vi "Dashboard Main.vi"() -> ()   [LabVIEW 2016]
uses:
  <vilib>/event_ctls.llb/eventvkey.ctl
  <vilib>/Utility/config.llb/NI_LVConfig.lvlib
  <vilib>/Utility/config.llb/Write Key (I32).vi
  <vilib>/Rock Robotics/WPI/Dashboard/WPI_DashboardLogging Global.vi
  <vilib>/Utility/config.llb/Write Key (String).vi
  <vilib>/Rock Robotics/Network Tables/NT Read Numeric Array.vi
  <vilib>/Utility/miscctls.llb/LVRowAndColumnTypeDef.ctl
  <vilib>/Instr/_visa.llb/VISA Configure Serial Port (Instr).vi
panel:
  in  "TCP":refnum<k5>
  in  "Rec Mode":enum32{"Stop", "Record", "Playback"}(radio)
  in  "Vision":u16(ring) items=["Camera Off", "USB Camera SW", "USB Camera HW", "IP Camera"]
  out "Camera IP":string
  out "Image Message":string="Timeout in Camera Communications"
  in  "Dashboard Tab":T1(tab)
  in  "Select Auto":string(combo)
  out "NT Connection":bool
  in  "Camera Settings":T2={"Frame Rate"=30, "Compression"=30, "Size"=1} {"Frame Rate" scale=1.0..30.0; "Size" items=["640x480", "320x240", "160x120"]}
  out "MotorChart R":cluster{"Numeric":dbl, "Numeric":dbl}(graph)
  out "MotorChart L":T3(graph)
  out "MotorSliders R":cluster{"MotorSlide1":dbl, "MotorSlide2":dbl} {"MotorSlide2" scale=-1.0..1.0 scale format="%#_2e"; "MotorSlide1" scale=-1.0..1.0 scale format="%#_2e"}
  out "MotorSliders L":T4 {"MotorSlide4 2" scale=0.0..14.0 scale format="%#_2e"; "MotorSlide2" scale=-1.0..1.0 scale format="%#_2e"; "MotorSlide1" scale=-1.0..1.0 scale format="%#_2e"}
  out "Gyro":dbl(knob) scale=0.0..360.0
  out "JS1 Z":dbl(slide) scale=-1.0..1.0 scale format="%#_2e"
  out "JS1 Graph":cluster{"X":dbl, "Y":dbl}[](graph)
  out "JS1 Buttons":T5
  out "JS2 Z":dbl(slide) scale=-1.0..1.0 scale format="%#_2e"
  out "JS2 Graph":cluster{"X":dbl, "Y":dbl}[](graph)
  out "JS2 Buttons":T5
  out "Mode":T6(ring)=enum."Auto Disabled"
  in  "DB Camera Config":bool
  out "fps":dbl format="%#.1g"
  out "Mbps":dbl format="%#.1g"
  out "Mbps LED":bool
  in  "DB/String 9":string
  in  "DB/String 8":string
  in  "DB/String 7":string
  in  "DB/String 6":string
  in  "DB/String 5":string
  in  "DB/String 4":string
  in  "DB/String 3":string
  in  "DB/String 2":string
  in  "DB/String 1":string
  in  "DB/String 0":string
  in  "DB/Slider 0":dbl(slide) scale=0.0..5.0
  in  "DB/Slider 1":dbl(slide) scale=0.0..5.0
  in  "DB/Slider 2":dbl(slide) scale=0.0..5.0
  in  "DB/Slider 3":dbl(slide) scale=0.0..5.0
  out "DB/LED 3":bool
  out "DB/LED 2":bool
  out "DB/LED 1":bool
  out "DB/LED 0":bool
  in  "DB/Button 3":bool
  in  "DB/Button 2":bool
  in  "DB/Button 1":bool
  in  "DB/Button 0":bool caption="New Name"
  out "Boolean":bool
  out "Gauge 2":u8(knob) scale=0.0..255.0
  out "Gauge":u8(knob) scale=0.0..255.0
  out "Boolean 3":bool
  in  "Boolean 2":bool
  out "String 2":string
  out "String":string
  in  "Boolean 4":bool
  out "Boolean 5":bool
  in  "Test Slider":dbl(slide) scale=0.0..100.0 scale format="%#_3g"
  in  "On/Off":bool caption="Solenoid"
  in  "Test Name":u16(ring) items=["Select the test to run..."]
  in  "Test Tree":string(tree)
  in  "Motor":cluster{"Value":dbl, "Enable":bool} {"Value" scale=-1.0..1.0 scale format="%#_3g"}
  out "Progress":T7 {"Test Progress" scale=0.0..100.0}
  in  "Rev/Fwd":cluster{"Forward":bool, "Reverse":bool}
  in  "Test Ring":u16(ring) items=["Monochrome", "Color"]
  out "Cmd Status":string
  in  "Execute Command":bool
  in  "Command Params":string[][](table)
  in  "Command Selection":i32(listbox)
  in  "CheckList":i32(listbox)
  out "Tree":string(tree)
  out "Camera Image":T8(plugin-control)
  out "Background":bool
  # "Left"
  # "Front"
  # "Right"
  # "Battery"
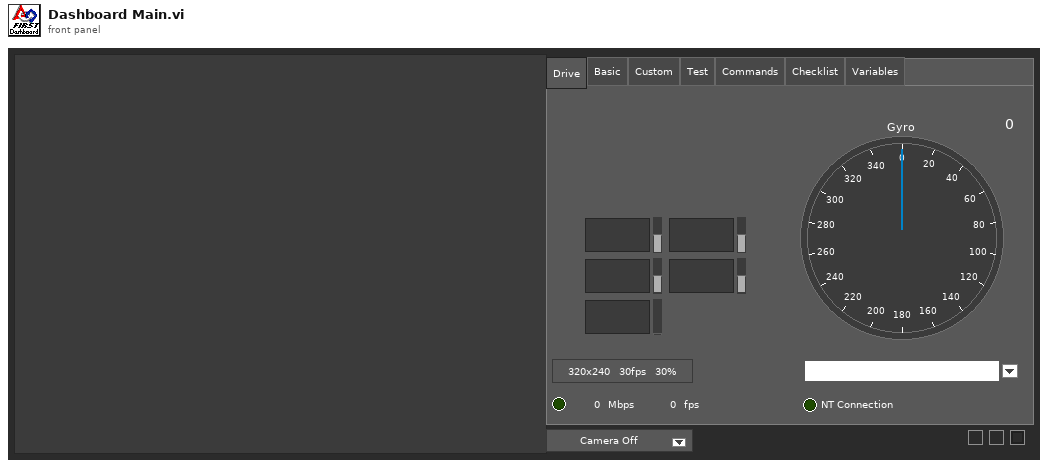
[diagram p1: front panel]
types:
  T1 = enum32{"Drive", "Basic", "Custom", "Test", "Commands", "Checklist", "Variables"}
  T2 = cluster{"Frame Rate":i32, "Compression":i32, "Size":u16}
  T3 = cluster{"Numeric":dbl, "Numeric":dbl, "Battery V":dbl}
  T4 = cluster{"MotorSlide1":dbl, "MotorSlide2":dbl, "MotorSlide4 2":dbl}
  T5 = cluster{bool, bool, bool, bool, bool, bool, bool, bool, bool, bool, bool, bool}
  T6 = enum8{"Tele-Op Disabled", "Tele-Op Enabled", "Auto Disabled", "Auto Enabled", "Test Disabled", "Test Enabled", "Disconnected", "No Code", "E-Stop"}
  T7 = cluster{"Test Progress":u8, "Test Progress Text":string}
  T8 = typedef "IMAQ Image.ctl" = refnum<image>
  T9 = cluster{"IDs":cluster{"RPC field ID":u16, "Unique ID":u16}, "String":string}
  T10 = enum32{"Drive", "Basic", "Custom", "Test", "Checklist", "Variables"}
  T11 = typedef "Image Type" = u32
  T12 = cluster{"Error Strings":string, "Disable Counts":cluster{u16, u16}, "Rail Faults":cluster{u16, u16, u16}, "Robot IP":string, "DB Mode":u8, "Event Info":cluster{"Name":string, "Type":u8, "Number":u16, "Replay":u8}}
  T13 = cluster{"Storage":cluster{"Disk Free":u64, "RAM Block":u32, "RAM free":u32}, "CPU Utilization":cluster{"CPU % ISR":sgl, "CPU % Time Crit":sgl, "CPU % Timed Str":sgl, "CPU % High":sgl, "CPU % Above":sgl, "CPU % Normal":sgl, "CPU % Low":sgl}, "CAN":cluster{"% Bus Utilization":sgl, "Bus Off Cnt":u32, "TX_FIFO Full Cnt":u32, "Receive Error Cnt":u8, "Transmit Error Cnt":u8}, "HID":cluster{"HID Outputs":u32, "Rumble Low":u16, "Rumble High":u16}[]}
  T14 = cluster{"Status bits":cluster{"Test Mode":bool, "Autonomous":bool, "Enabled":bool, "Code Start":bool, "Brownout":bool, "Reserved 2":bool, "Reserved 3":bool, "E-Stop":bool}, "Code Trace":cluster{"Disabled":bool, "TeleOp":bool, "Auto":bool, "Test":bool}, "Controller Type":enum16{"unknown", "cRIO", "roboRio"}, "Code?":enum16{"unknown", "noCode", "code"}, "Battery V":dbl}
  T15 = cluster{"Control Bits":cluster{"TestMode":bool, "Autonomous":bool, "Enabled":bool, "FMS Present":bool, bool, bool, bool, "E-Stop":bool}, "Team Station ":u8, "Countdown":sgl, "Joystick Values":cluster{"Axes":dbl[], "Buttons":bool[], "POVs":i16[]}[]}
  T16 = cluster{"Axes":dbl[], "Buttons":bool[], "POVs":i16[]}[]
  T17 = cluster{"Axes":dbl[], "Buttons":bool[], "POVs":i16[]}
  T18 = cluster{"Buttons[0]":bool, "Buttons[1]":bool, "Buttons[2]":bool, "Buttons[3]":bool, "Buttons[4]":bool, "Buttons[5]":bool, "Buttons[6]":bool, "Buttons[7]":bool, "Buttons[8]":bool, "Buttons[9]":bool, "Buttons[10]":bool, "Buttons[11]":bool}
  T19 = cluster{"Camera Image":refnum<vi>, "Dashboard Tab":refnum<vi>, "Background":refnum<vi>, "Vision":refnum<vi>, "Rec Mode":refnum<vi>, "Test Slider":refnum<vi>, "On/Off ":refnum<vi>, "Test Ring":refnum<vi>, "Rev/Fwd":refnum<vi>, "Test Name":refnum<vi>, "Motor":refnum<vi>, "Progress":refnum<vi>, "CheckList":refnum<vi>, "Tree":refnum<vi>, "Test Tree":refnum<vi>, "Command Params":refnum<vi>, "Command Selection":refnum<vi>, "Execute Command":refnum<vi>, "Cmd Status":refnum<vi>}
  T20 = typedef "NI_LVConfig.lvlib/Config Data RefNum.ctl" = refnum<k1>
  T21 = cluster{"Operation":enum16{"Update", "Clear"}, "Color Box":u32}[]
  T22 = typedef "eventvkey.ctl" = enum16{"ASCII", "Enter", "Return", "Shift", "Ctrl", "Alt", "Cmd", "Opt", "Caps", "NumLock", "Clear", "Break", "Up", "Down", "Left", "Right", "Insert", "Delete", "Home", "End", "PageUp", "PageDown", "Escape", "Help", "Pause", "ScrollLock", "F1", "F2", "F3", "F4", "F5", "F6", "F7", "F8", "F9", "F10", "F11", "F12", "F13", "F14", "F15", "F16", "F17", "F18", "F19", "F20", "F21", "F22", "F23", "F24", "Play", "VolumeUp", "VolumeDown", "Mute", "Two Byte Char"}
  T23 = cluster{"Image Size":bool, "Image Type":bool, "Pixel Value":bool, "ROI Information":bool, "Zoom Factor":bool}
  T24 = enum8{"Enabled", "Disabled", "Disabled and Grayed Out"}
  T25 = cluster{"Operation":enum16{"Update", "Clear"}, "Color Box":u32}
  T26 = typedef "LVRowAndColumnTypeDef.ctl" = cluster{"Row":i32, "Column":i32}
  T27 = cluster{"Shift":bool, "Ctrl":bool, "Alt":bool, "Cmd":bool, "Opt":bool}
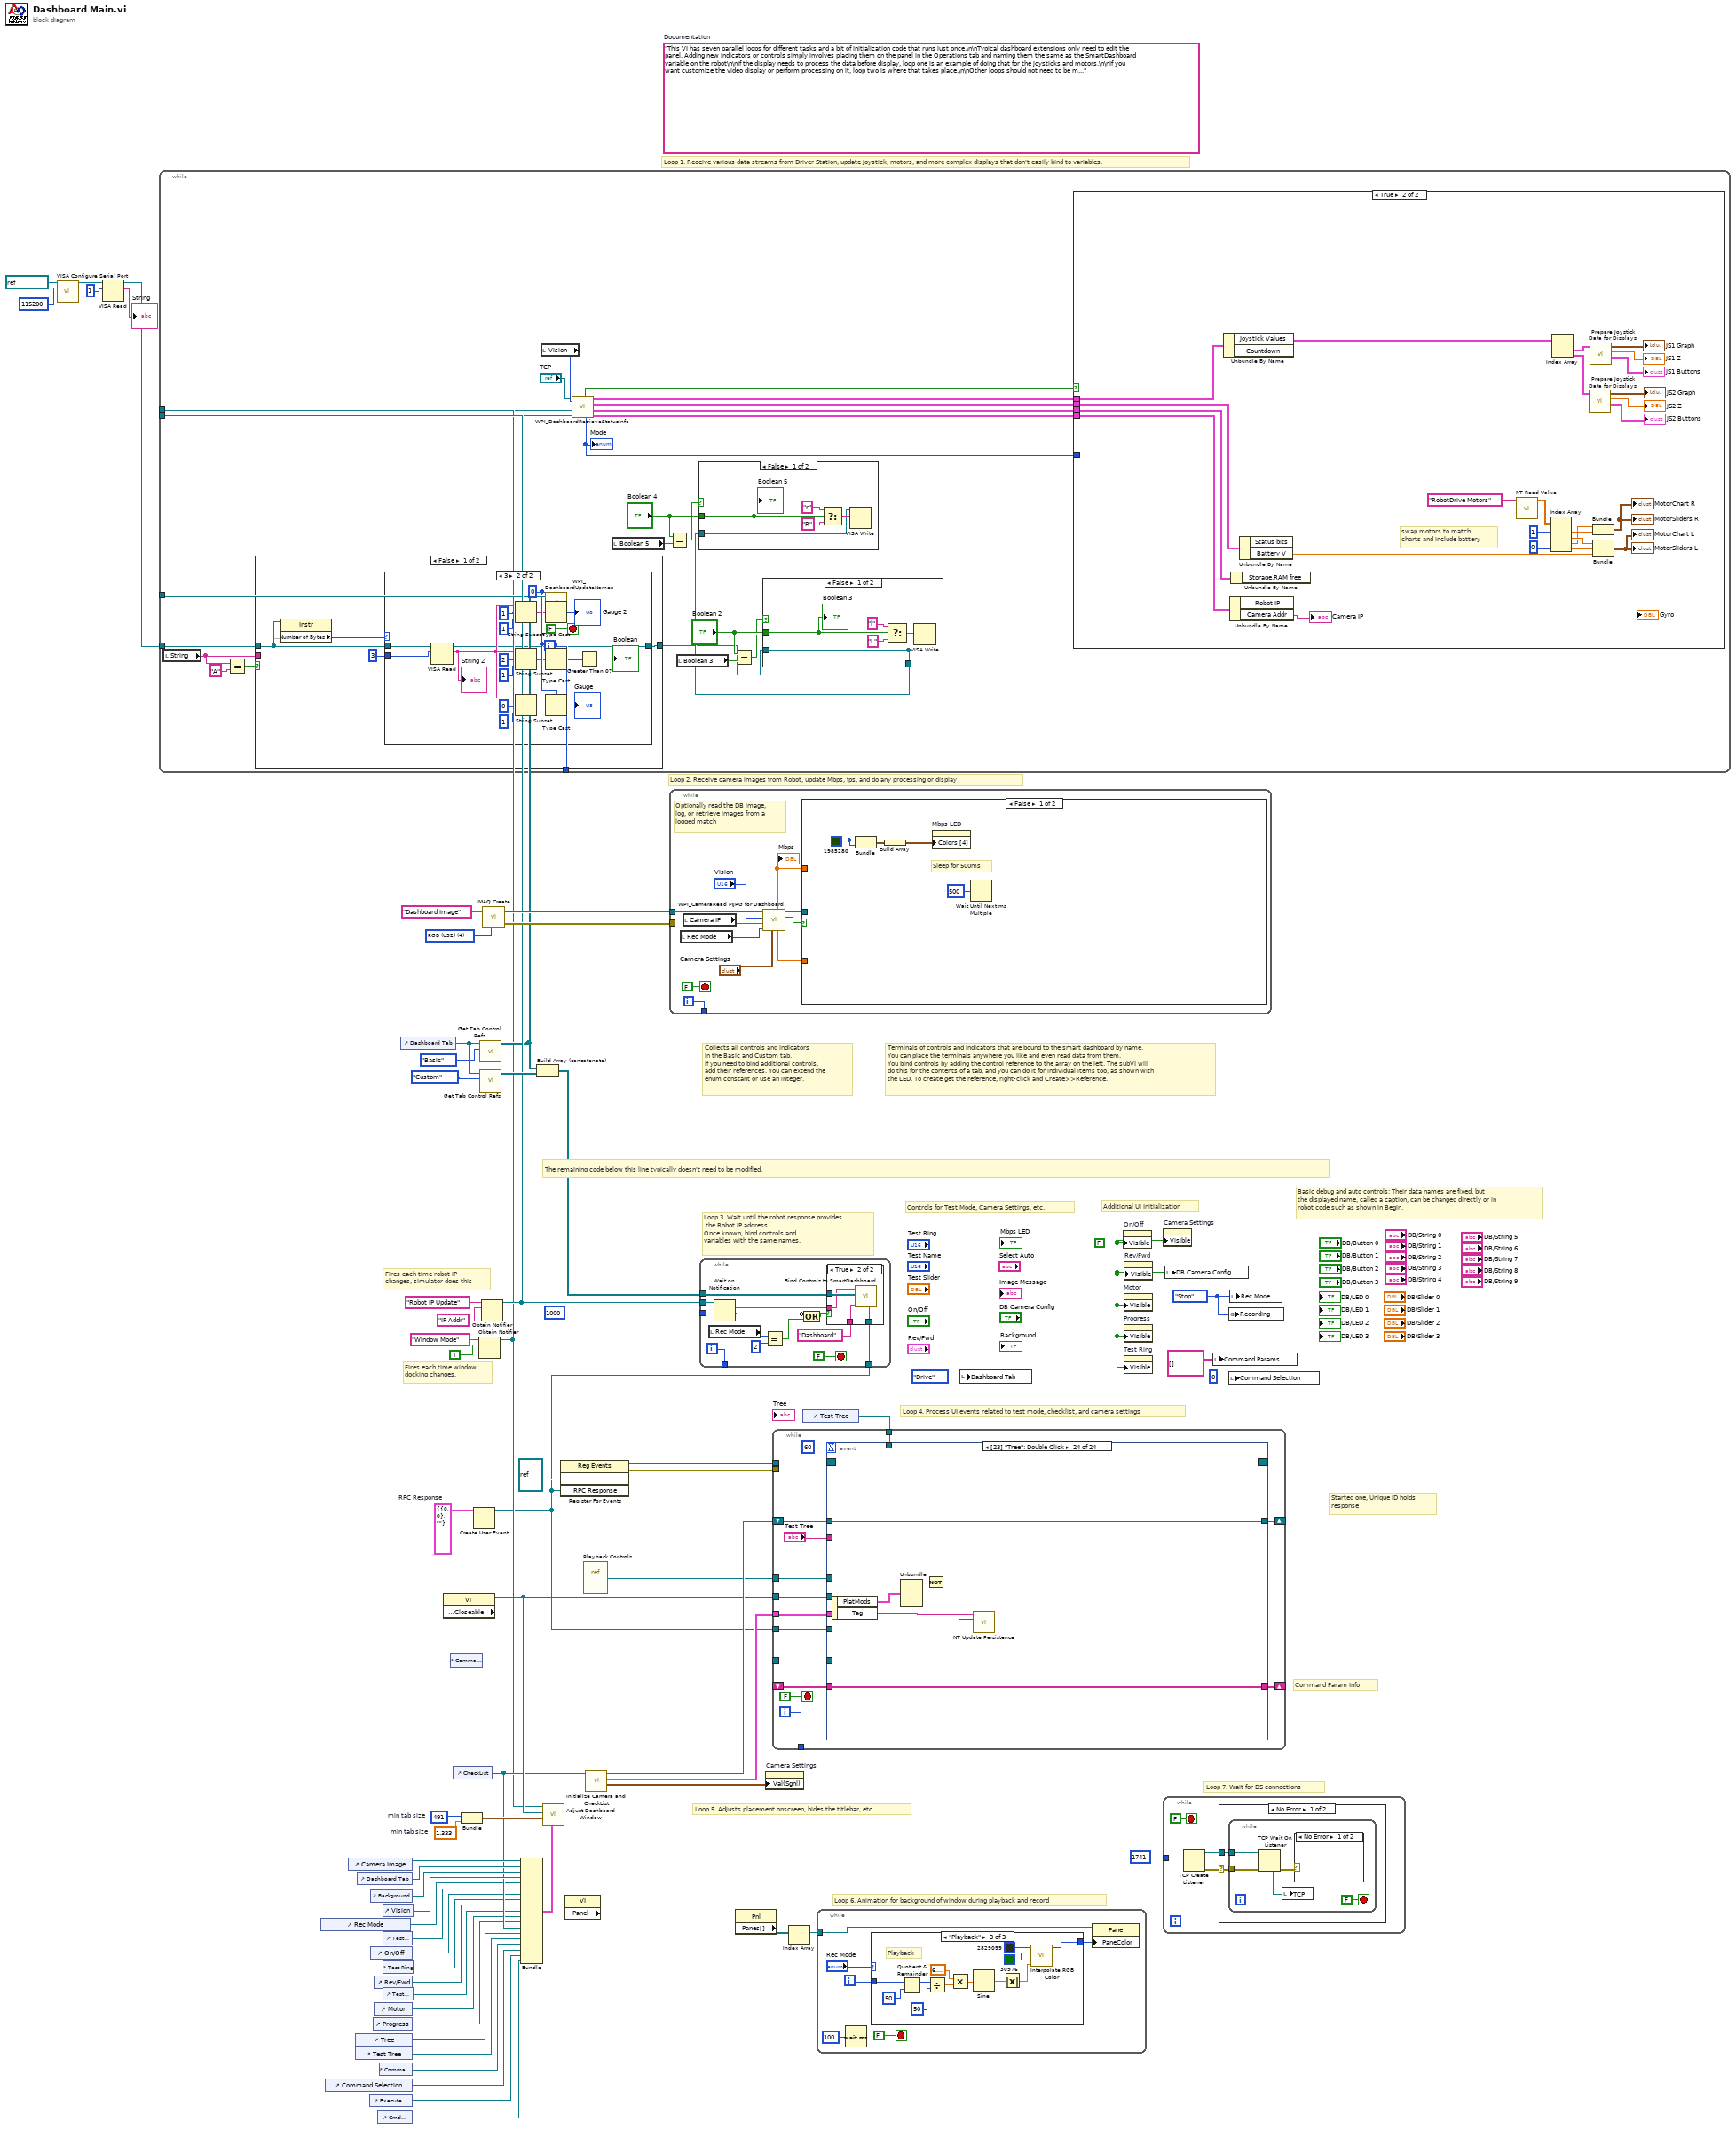
[diagram p0: block diagram]
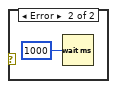
[diagram p2: hidden frame]
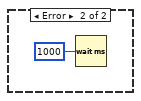
[diagram p3: hidden frame]
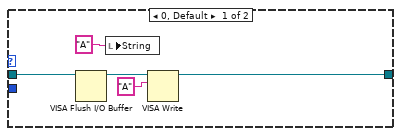
[diagram p6: hidden frame]
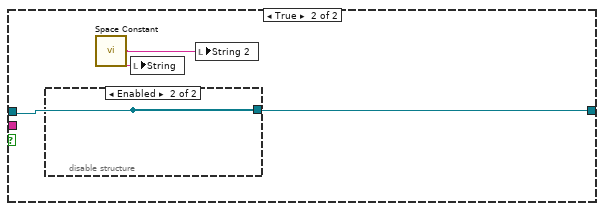
[diagram p7: hidden frame]
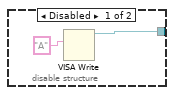
[diagram p8: hidden frame]
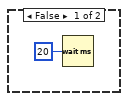
[diagram p9: hidden frame]
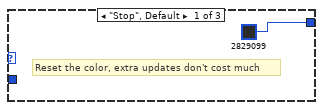
[diagram p10: hidden frame]
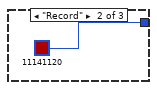
[diagram p11: hidden frame]
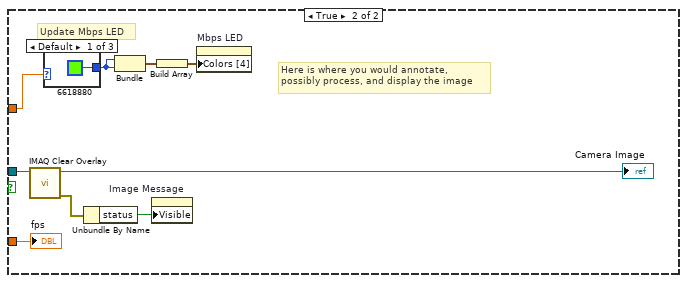
[diagram p13: hidden frame]
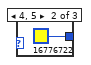
[diagram p14: hidden frame]
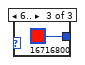
[diagram p15: hidden frame]
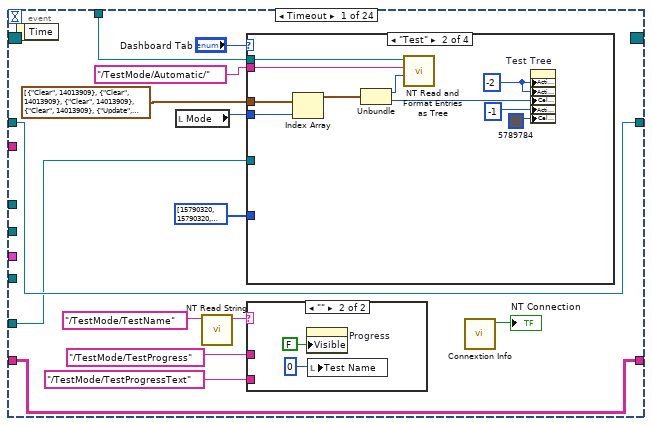
[diagram p16: hidden frame]
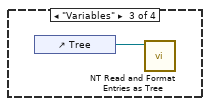
[diagram p18: hidden frame]
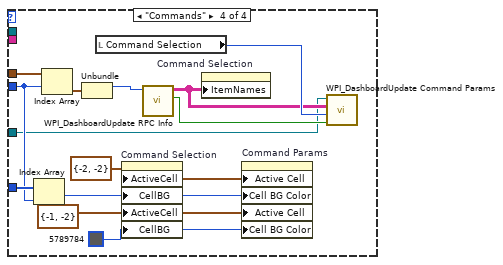
[diagram p19: hidden frame]
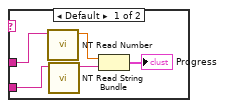
[diagram p20: hidden frame]
diagram:
  w13 = T9 {"IDs"={"RPC field ID"=0, "Unique ID"=0}, "String"=""}  # RPC Response
  w39 = 491  # min tab size
  w38 = 1.333  # min tab size
  w47 = enum32{"Stop", "Record", "Playback"}."Stop" ("Rec Mode")
  w21 = FALSE ("Visible")
  (unwired) "This VI has seven parallel loops for different tasks and a bit of initialization code that runs just once.\n\nTypical dashboard extensions only need to edit the panel. Adding new indicators or controls simply involves placing them on the panel in the Operations tab and naming them the same as the SmartDashboard variable on the robot\n\nIf the display needs to process the data before display, loop one is an example of doing that for the joysticks and motors.\n\nIf you want customize the video display or perform processing on it, loop two is where that takes place.\n\nOther loops should not need to be modified. They are pretty standard, and document the task they perform."  # Documentation
  w67 = T11 4 items=["Grayscale (U8)", "Grayscale (I16)", "Grayscale (SGL)", "Complex (CSG)", "RGB (U32)", "HSL (U32)", "RGB (U64)"] ("Image Type")
  # "Command Param Info"
  # "Started one, Unique ID holds\nresponse"
  # "Loop 7. Wait for DS connections"
  # "Basic debug and auto controls: Their data names are fixed, but\nthe displayed name, called a caption, can be changed directly or in\nrobot code such as shown in Begin."
  # "Controls for Test Mode, Camera Settings, etc."
  # "Additional UI Initialization"
  # "Loop 6. Animation for background of window during playback and record"
  # "Fires each time robot IP\nchanges, simulator does this"
  # "Fires each time window\ndocking changes."
  # "Collects all controls and indicators\nin the Basic and Custom tab.\nIf you need to bind additional controls,\nadd their references. You can extend the\nenum constant or use an integer."
  # "The remaining code below this line typically doesn't need to be modified."
  # "Loop 4. Process UI events related to test mode, checklist, and camera settings"
  # "Terminals of controls and indicators that are bound to the smart dashboard by name.\nYou can place the terminals anywhere you like and even read data from them.\nYou bind controls by adding the control reference to the array on the left. The subVI will\ndo this for the contents of a tab, and you can do it for individual items too, as shown with\nthe LED. To create get the reference, right-click and Create>>Reference."
  # "Loop 3. Wait until the robot response provides\n the Robot IP address.\nOnce known, bind controls and\nvariables with the same names."
  # "Loop 5. Adjusts placement onscreen, hides the titlebar, etc."
  # "Loop 1. Receive various data streams from Driver Station, update joystick, motors, and more complex displays that don't easily bind to variables."
  # "Loop 2. Receive camera images from Robot, update Mbps, fps, and do any processing or display"
  n1 = call-poly "VISA Configure Serial Port"("VISA resource name"=refnum<visa-resource-name> "COM5", "baud rate (9600)"=u32 115200) -> ("VISA resource name out"=w3:refnum<visa-resource-name>)  [unwired: 12 in, 1 out]
  n2 = VISA Read(VISA resource name=w3, byte count=u32 1) -> (VISA resource name out=w1:refnum<visa-resource-name>, read buffer=→"String":string)  [unwired: 1 in, 2 out]
  n3 = control-ref of="Rec Mode"() -> (w27:refnum<vi>)
  n4 = control-ref of="Command Selection"() -> (w12:refnum<vi>)
  n5 = control-ref of="Camera Image"() -> (w42:refnum<vi>)
  n6 = control-ref of="Tree"() -> (w31:refnum<vi>)
  n7 = control-ref of="Test Tree"() -> (w30:refnum<vi>)
  n8 = control-ref of="Dashboard Tab"() -> (w41:refnum<vi>)
  n9 = control-ref of="Execute Command"() -> (w14:refnum<vi>)
  n10 = control-ref of="Background"() -> (w36:refnum<vi>)
  n11 = control-ref of="On/Off"() -> (w25:refnum<vi>)
  n12 = control-ref of="Progress"() -> (w22:refnum<vi>)
  n13 = control-ref of="Rev/Fwd"() -> (w23:refnum<vi>)
  n14 = control-ref of="Motor"() -> (w28:refnum<vi>)
  n15 = control-ref of="Cmd Status"() -> (w8:refnum<vi>)
  n16 = control-ref of="Command Params"() -> (w15:refnum<vi>)
  n17 = control-ref of="Test Slider"() -> (w26:refnum<vi>)
  n18 = control-ref of="Vision"() -> (w40:refnum<vi>)
  n19 = control-ref of="Test Ring"() -> (w24:refnum<vi>)
  n20 = control-ref of="Test Name"() -> (w29:refnum<vi>)
  n21 = control-ref of="Dashboard Tab"() -> (w45:refnum<vi>)
  n22 = property class="VI" props=["Front Panel.Closeable"]() -> (reference out=w46:refnum<vi>)  [unwired: 2 in, 2 out]
  n23 = control-ref of="Command Params"() -> (w7:refnum<vi>)
  n24 = control-ref of="CheckList"() -> (w32:refnum<vi>)
  n25 = Bundle("min tab size"=w39, "min tab size"=w38) -> (w37:cluster{"min tab size":i32, "min tab size":dbl})  [unwired: 1 in]
  n26 = Create User Event(user event datatype=w13) -> (user event=w9:refnum<user-event>)  [unwired: 1 in, 1 out]
  n27 = Obtain Notifier(name (unnamed)="Window Mode", notification data type=TRUE) -> (notifier out=w18:refnum<notifier>)  [unwired: 2 in, 2 out]
  n28 = call <vilib>:"Get Tab Control Refs.vi"("Page Index"=T10."Basic" ("Dashboard Tab"), "TabControl in"=w45) -> ("ControlsOnPage"=w19:refnum<vi>[])  [unwired: 9 in]
  n29 = call <vilib>:"Get Tab Control Refs.vi"("Page Index"=T10."Custom" ("Dashboard Tab"), "TabControl in"=w45) -> ("ControlsOnPage"=w44:refnum<vi>[])  [unwired: 9 in]
  n30 = Obtain Notifier(name (unnamed)="Robot IP Update", notification data type="IP Addr" ("name (unnamed)")) -> (notifier out=w20:refnum<notifier>)  [unwired: 2 in, 2 out]
  n31 = while {
    tunnel: [w91] -> _
    tunnel: w20 -> [w85]
    tunnel: w19 -> [w84]
    tunnel: w18 -> [w80]
    tunnel: w1 -> [w73]
    i -> [w91]
    stop <- FALSE stop-if-true
    n32 = local read "String"() -> (w76:string)
    n33 = Equal?(x=w76, y="A") -> (x = y?=w75:bool)
    n34 = case shown="False" w75 {
      tunnel: w73 -> [w106 w131]
      tunnel: w76 -> [_ _]
      tunnel: [w104 w131] -> w68
      frame False {
        n35 = property class="Instr"(reference=w106) -> ("Serial Settings:Number of Bytes at Serial Port"=w105:u32)  [unwired: 1 in, 2 out]
        n36 = case shown="3" w105 {
          tunnel: u32 3 ("byte count") -> [_ w128]
          tunnel: w106 -> [w111 w127]
          tunnel: [w108 w113] -> w104
          frame 0, Default {
            n37 = VISA Flush I/O Buffer(VISA resource name=w111) -> (VISA resource name out=w109:refnum<visa-resource-name>)  [unwired: 2 in, 1 out]
            n38 = local write "String"("A" ("String")) -> ()
            n39 = VISA Write(VISA resource name=w109, write buffer="A") -> (VISA resource name out=w108:refnum<visa-resource-name>)  [unwired: 1 in, 2 out]
          }
          frame 3 {
            w129 = u8 0
            n40 = VISA Read(VISA resource name=w127, byte count=w128) -> (VISA resource name out=w113:refnum<visa-resource-name>, read buffer=w116:string)  [unwired: 1 in, 2 out]
            "String 2" <- w116
            n41 = String Subset(string=w116, offset (0)=1, length (rest)=1 ("length (rest)")) -> (substring=w115:string)
            n42 = String Subset(string=w116, offset (0)=2, length (rest)=1 ("length (rest)")) -> (substring=w121:string)
            n43 = String Subset(string=w116, offset (0)=0, length (rest)=1 ("length (rest)")) -> (substring=w114:string)
            n44 = Type Cast(type=w129, x=w115) -> (*(type *) &x=→"Gauge 2":u8)
            n45 = Type Cast(type=w129, x=w121) -> (*(type *) &x=w125:u8)
            n46 = Type Cast(type=w129, x=w114) -> (*(type *) &x=→"Gauge":u8)
            n47 = Greater Than 0?(x=w125) -> (x > 0?=→"Boolean":bool)
          }
        }
      }
      frame True {
        n48 = disable-structure shown="Enabled" {
          disable-tunnel: w131 -> [w133 _]
          frame Disabled {
            n49 = VISA Write(VISA resource name=w133, write buffer="A") -> ()  [unwired: 1 in, 3 out]
          }
          frame Enabled {
          }
        }
        n50 = call <vilib>:"Space Constant.vi"() -> ("String"=w132:string)
        n51 = local write "String"(w132) -> ()
        n52 = local write "String 2"(w132) -> ()
      }
    }
    n53 = local read "Vision"() -> (w82:u16)
    n54 = call <vilib>:"WPI_DashboardUpdateNames.vi"("Controls on Tab"=w84) -> ()  [unwired: 11 in]
    n55 = call <vilib>:"WPI_DashboardRetrieveStatusInfo.vi"(7:w82, "Binding Refnum"=w85, "Window Mode Notifier"=w80, "TCP Cnx"="TCP") -> ("Power and Errors"=w86:T12, "Robot Metrics"=w89:T13, "Status Info"=w90:T14, "Control Info"=w87:T15, "Robot Mode"=w83:T6, "Process?"=w88:bool)  [unwired: 2 in]
    "Mode" <- w83
    n56 = local read "Boolean 5"() -> (w70:bool)
    n57 = Equal?(x="Boolean 4", y=w70) -> (x = y?=w71:bool)
    n58 = local read "Boolean 3"() -> (w77:bool)
    n59 = Equal?(x="Boolean 2", y=w77) -> (x = y?=w78:bool)
    n60 = case shown="False" w78 {
      tunnel: "Boolean 2" -> [w100 _]
      tunnel: w68 -> [w98 w103]
      tunnel: [w98 w103] -> w69
      frame False {
        n61 = Select(t="l" ("write buffer"), s=w100, f="L" ("write buffer")) -> (s? t:f=w99:string)
        n62 = VISA Write(VISA resource name=w98, write buffer=w99) -> ()  [unwired: 1 in, 3 out]
        "Boolean 3" <- w100
      }
      frame True {
      }
    }
    n63 = case shown="False" w71 {
      tunnel: "Boolean 4" -> [w95 _]
      tunnel: w69 -> [w93 _]
      frame False {
        n64 = Select(t="r" ("write buffer"), s=w95, f="R" ("write buffer")) -> (s? t:f=w94:string)
        n65 = VISA Write(VISA resource name=w93, write buffer=w94) -> ()  [unwired: 1 in, 3 out]
        "Boolean 5" <- w95
      }
      frame True {
      }
    }
    n66 = case shown="True" w88 {
      tunnel: w90 -> [_ w160]
      tunnel: w89 -> [_ w159]
      tunnel: w87 -> [_ w158]
      tunnel: w86 -> [_ w157]
      tunnel: w83 -> [_ _]
      frame False {
        n67 = Wait (ms)(milliseconds to wait=u32 20) -> ()  [unwired: 1 out]
      }
      frame True {
        # "swap motors to match\ncharts and include battery"
        n68 = Unbundle By Name(w158) -> ("Joystick Values"=w147:T16)  [unwired: 1 out]
        n69 = Unbundle By Name(w157) -> ("Camera Addr"=→"Camera IP":string)  [unwired: 1 out]
        n70 = Unbundle By Name(w159) -> ()  [unwired: 1 out]
        n71 = Unbundle By Name(w160) -> ("Battery V"=w148:dbl)  [unwired: 1 out]
        n72 = call-poly <vilib>:"NT Read Value.vi"("Name"="RobotDrive Motors") -> ("Numeric Array"=w136:dbl[])  [unwired: 9 in, 1 out]
        n73 = Index Array(array=w136, index #1=1, index #4=0) -> (element #1=w152:dbl, element #2=w153:dbl, element #3=w151:dbl, element #4=w156:dbl)  [unwired: 2 in]
        n74 = Index Array(array=w147) -> (element #1=w146:T17, element #2=w141:T17)  [unwired: 2 in]
        n75 = call "Prepare Joystick Data for Displays.vi"("Joystick Values"=w141) -> ("Buttons"=→"JS2 Buttons":T18, "Z Axis"=→"JS2 Z":dbl, "Cartesian Data"=→"JS2 Graph":cluster{"X axis":dbl, "X axis":dbl}[])  [unwired: 8 in]
        n76 = call "Prepare Joystick Data for Displays.vi"("Joystick Values"=w146) -> ("Buttons"=→"JS1 Buttons":T18, "Z Axis"=→"JS1 Z":dbl, "Cartesian Data"=→"JS1 Graph":cluster{"X axis":dbl, "X axis":dbl}[])  [unwired: 8 in]
        n77 = Bundle("Numeric"=w151, "Numeric"=w152) -> (→"MotorChart R" →"MotorSliders R":cluster{"Numeric":dbl, "Numeric":dbl})  [unwired: 1 in]
        n78 = Bundle("Numeric"=w153, "Numeric"=w156, "Battery V"=w148) -> (→"MotorChart L" →"MotorSliders L":T3)  [unwired: 1 in]
      }
    }
  }
  n79 = call "IMAQ Create"("Image Name"="Dashboard Image", "Image Type"=w67) -> ("New Image"=w65:T8, "error out"=w64:errorcluster)  [unwired: 2 in, 1 out]
  n80 = Bundle("Camera Image"=w42, "Dashboard Tab"=w41, "Background"=w36, "Vision"=w40, "Rec Mode"=w27, "Test Slider"=w26, "On/Off"=w25, "Test Ring"=w24, "Rev/Fwd"=w23, "Test Name"=w29, "Motor"=w28, "Progress"=w22, "CheckList"=w32, "Tree"=w31, "Test Tree"=w30, "Command Params"=w15, "Command Selection"=w12, "Execute Command"=w14, "Cmd Status"=w8) -> (w33:T19)  [unwired: 1 in]
  n81 = Build Array (concatenate)(w19, w44) -> (w43:refnum<vi>[])
  n82 = call "Adjust Dashboard Window.vi"("Sizing Refnums"=w33, "Size Constraints"=w37, "VI"=w46, "WIn Mode"=w18) -> ()  [unwired: 8 in]
  n83 = register-events(refnum<vi> refnum, w9) -> (reference out=w51:refnum<event-registration>, error out=w50:errorcluster)  [unwired: 2 in]
  n84 = property class="VI"() -> ("Panel"=w54:refnum<vi>)  [unwired: 2 in, 2 out]
  n85 = vi-ref "Playback Controls.vi"() -> (w52:refnum<vi>)
  n86 = call "Initialize Camera and CheckList.vi"("ListBox in"=w32) -> ("Cluster"=w58:cluster{"value":i32, "value":i32, "index":i32}, "Array"=w59:cluster{string[]}[], "File Refnum"=w57:T20)  [unwired: 8 in]
  n87 = while {
    tunnel: w65 -> [w169]
    tunnel: w64 -> [_]
    tunnel: [w170] -> _
    i -> [w170]
    stop <- FALSE stop-if-true
    # "Optionally read the DB image,\nlog, or retrieve images from a\nlogged match"
    n88 = local read "Rec Mode"() -> (w164:enum32{"Stop", "Record", "Playback"})
    n89 = local read "Camera IP"() -> (w162:string)
    n90 = call <vilib>:"WPI_CameraRead MJPG for Dashboard.vi"("Camera Settings"="Camera Settings", "Rec Mode"=w164, "Robot IP"=w162, "Camera Name"="Vision", "Refnum in"=w169) -> ("Active"=w167:bool, "Refnum out"=w168:T8, "FPS"=w166:dbl, "Bandwidth (Mbps)"=w161:dbl)  [unwired: 3 in]
    "Mbps" <- w161
    n91 = case shown="False" w167 {
      tunnel: w168 -> [_ w179]
      tunnel: w161 -> [_ w178]
      tunnel: w166 -> [_ w176]
      frame False {
        w172 = u32 1985280 ("Color Box")
        # "Sleep for 500ms"
        n92 = Bundle("Color Box"=w172, "Color Box"=w172) -> (w174:cluster{"Color Box":u32, "Color Box":u32})  [unwired: 1 out]
        n93 = Build Array(w174) -> (w173:cluster{"Color Box":u32, "Color Box":u32}[])
        n94 = property on="Mbps LED" class="Bool (strict)"("Colors [4]"=w173) -> ()  [unwired: 2 in, 2 out]
        n95 = Wait Until Next ms Multiple(millisecond multiple=u32 500) -> ()  [unwired: 1 out]
      }
      frame True {
        # "Here is where you would annotate,\npossibly process, and display the image"
        # "Update Mbps LED"
        n96 = call "IMAQ Clear Overlay"("Image"=w179) -> ("error out"=w183:errorcluster, "Image Out"=→"Camera Image":T8)  [unwired: 2 in, 7 out]
        n97 = case shown="Default" w178 {
          tunnel: [u32 6618880 ("Color Box") u32 16776722 ("Color Box") u32 16716800 ("Color Box")] -> w180
          frame Default {
          }
          frame 4, 5 {
          }
          frame 6.. {
          }
        }
        n98 = Unbundle By Name(w183) -> ("status"=w184:bool)
        n99 = Bundle("Color Box"=w180, "Color Box"=w180) -> (w182:cluster{"Color Box":u32, "Color Box":u32})  [unwired: 1 out]
        n100 = property on="Image Message" class="Str"("Visible"=w184) -> ()  [unwired: 2 in, 2 out]
        n101 = Build Array(w182) -> (w181:cluster{"Color Box":u32, "Color Box":u32}[])
        n102 = property on="Mbps LED" class="Bool (strict)"("Colors [4]"=w181) -> ()  [unwired: 2 in, 2 out]
        "fps" <- w176
      }
    }
  }
  n103 = while {
    tunnel: w43 -> [w200]
    tunnel: w20 -> [w198]
    tunnel: [w196] -> _
    tunnel: u32 1000 ("milliseconds to wait") -> [w195]
    tunnel: w9 -> [w188]
    i -> [w196]
    stop <- FALSE stop-if-true
    n104 = local read "Rec Mode"() -> (w191:enum32{"Stop", "Record", "Playback"})
    n105 = Wait on Notification(notifier=w198, timeout in ms (-1)=w195) -> (notification=w197:string, timed out?=w193:bool)  [unwired: 2 in, 2 out]
    n106 = Equal?(x=w191, y=u16 2 ("Rec Mode")) -> (x = y?=w192:bool)
    n107 = Compound Arithmetic op=OR(invert w193, w192) -> (w194:bool)
    n108 = case shown="True" w194 {
      tunnel: w200 -> [_ w204]
      tunnel: w197 -> [_ w203]
      tunnel: "Dashboard" -> [_ w202]
      tunnel: w188 -> [_ w201]
      frame False {
      }
      frame True {
        n109 = call <vilib>:"Bind Controls to SmartDashboard.vi"("RPC ref"=w201, "Client Name"=w202, "Bound Control Refs"=w204, "Server IP Address"=w203) -> ()  [unwired: 8 in]
      }
    }
  }
  n110 = property class="Pnl"(reference=w54) -> ("Panes[]"=w55:refnum<vi>[])  [unwired: 1 in, 2 out]
  n111 = property on="Camera Settings" class="Clust (strict)"("Val(Sgnl)"=w58) -> ()  [unwired: 2 in, 2 out]
  n112 = Index Array(array=w55) -> (element=w53:refnum<vi>)  [unwired: 1 in]
  n113 = control-ref of="Test Tree"() -> (w56:refnum<vi>)
  n114 = while {
    tunnel: w59 -> [w216]
    shift-right: [w215] -> _
    shift-left: w57 -> [w214]
    tunnel: [w213] -> _
    tunnel: w56 -> [w212]
    tunnel: w52 -> [w211]
    tunnel: w51 -> [w210]
    tunnel: w50 -> [_]
    tunnel: w46 -> [w209]
    tunnel: w9 -> [w208]
    tunnel: w7 -> [w207]
    shift-right: [w206] -> _
    shift-left: _ -> [w205]
    i -> [w213]
    stop <- FALSE stop-if-true
    n115 = event shown="[23] \"Tree\": Double Click" {
      selector: w210 -> [_ _ _ _ _ _ _ _ _ _ _ _ _ _ _ _ _ _ _ _ _ _ _ _]
      dyn-events: [_ _ _ _ _ _ _ _ _ _ _ _ _ _ _ _ _ _ w525 _ _ _ _ _] -> _
      timeout: u32 60 ("milliseconds to wait") -> [_ _ _ _ _ _ _ _ _ _ _ _ _ _ _ _ _ _ _ _ _ _ _ _]
      tunnel: w212 -> [w229 _ _ _ _ _ _ _ _ _ _ _ _ _ _ _ _ _ _ _ _ _ _ _]
      tunnel: "Test Tree" -> [_ _ _ _ _ _ _ _ _ _ _ _ _ w488 w497 w500 w505 w514 _ _ _ _ _ _]
      tunnel: w216 -> [_ w267 _ _ _ _ _ _ _ _ _ w450 w481 _ _ _ _ _ _ _ _ _ _ _]
      tunnel: [w226 w266 w370 w376 w386 w390 w396 w408 w416 w422 w435 w449 w474 w487 w495 w499 w504 w513 w527 w543 w545 w553 w564 w569] -> w215
      tunnel: w214 -> [w226 w266 w370 w376 w386 w390 w396 w408 w416 w422 w435 w448 w474 w487 w495 w499 w504 w513 w527 w543 w545 w553 w564 w569]
      tunnel: w211 -> [_ _ _ _ _ _ _ _ _ _ _ _ _ _ _ _ _ _ w528 _ w548 _ _ _]
      tunnel: w209 -> [_ _ _ _ _ _ _ _ _ _ _ _ _ _ _ _ _ _ w523 _ _ _ _ _]
      tunnel: w208 -> [_ _ _ _ _ _ _ _ _ _ _ _ _ _ _ _ _ _ w519 _ _ _ _ _]
      tunnel: w207 -> [w221 _ _ _ _ _ w394 _ _ _ _ _ _ _ _ _ _ _ _ _ _ _ _ _]
      tunnel: [w220 w265 w369 w375 w385 w391 w392 w402 w413 w421 w434 w447 w473 w486 w494 w498 w503 w512 w518 w541 w544 w549 w557 w570] -> w206
      tunnel: w205 -> [w220 w265 w369 w375 w385 w391 w392 _ _ w421 w434 w447 w473 w486 w494 w498 w503 w512 w518 w541 w544 w549 w557 w570]
      event Timeout {
        n116 = event-data() -> ()  [unwired: 1 in, 1 out]
        n117 = local read "Mode"() -> (w223:T6)
        n118 = call <vilib>:"NT Read String.vi"("Name"="/TestMode/TestName") -> ("String"=w232:string)  [unwired: 9 in, 1 out]
        n119 = case shown="\"Test\"" "Dashboard Tab" {
          tunnel: w229 -> [_ w243 _ _]
          tunnel: "/TestMode/Automatic/" ("Name Pattern") -> [_ w242 _ _]
          tunnel: T21 [{"Operation"=enum."Clear", "Color Box"=14013909}, {"Operation"=enum."Clear", "Color Box"=14013909}, {"Operation"=enum."Clear", "Color Box"=14013909}, {"Operation"=enum."Clear", "Color Box"=14013909}, {"Operation"=enum."Update", "Color Box"=14013909}, {"Operation"=enum."Update", "Color Box"=16777215}, {"Operation"=enum."Clear", "Color Box"=14013909}, {"Operation"=enum."Clear", "Color Box"=14013909}, {"Operation"=enum."Clear", "Color Box"=14013909}] -> [_ w235 _ w252]
          tunnel: w223 -> [_ w234 _ w251]
          tunnel: u32[] [15790320, 15790320, 15790320, 15790320, 16777215, 16777215, 15790320, 15790320, 15790320] -> [_ _ _ w257]
          tunnel: w221 -> [_ _ _ w245]
          frame "Custom", Default {
          }
          frame "Test" {
            w241 = -2 ("Active Item:Row Number")
            n120 = Index Array(array=w235, index=w234) -> (element=w236:T25)
            n121 = Unbundle(w236) -> ("Operation"=w237:enum16{"Update", "Clear"}, "Color Box"=w238:u32)
            n122 = call <vilib>:"NT Read and Format Entries as Tree.vi"("Operation"=w237, "Name Pattern"=w242, "Tree Refnum"=w243) -> ()  [unwired: 7 in, 2 out]
            n123 = property on="Test Tree" class="Tree (strict)"("Active Item Row Number"=w241, "ActiveColNum"=w241, "CellBG"=w238, "Active Item Row Number"=-1 ("Active Item:Row Number"), "CellBG"=u32 5789784 ("Color Box")) -> ()  [unwired: 2 in, 2 out]
          }
          frame "Variables" {
            n124 = control-ref of="Tree"() -> (w244:refnum<vi>)
            n125 = call <vilib>:"NT Read and Format Entries as Tree.vi"("Tree Refnum"=w244) -> ()  [unwired: 9 in, 2 out]
          }
          frame "Commands" {
            w253 = u32 5789784 ("Color Box")
            w254 = T26 {"Row"=-1, "Column"=-2} ("Active Cell:Active Cell")
            w256 = T26 {"Row"=-2, "Column"=-2} ("Active Cell:Active Cell")
            n126 = Index Array(array=w257, index=w251) -> (element=w255:u32)
            n127 = Index Array(array=w252, index=w251) -> (element=w250:T25)
            n128 = Unbundle(w250) -> ("Operation"=w249:enum16{"Update", "Clear"})  [unwired: 1 out]
            n129 = local read "Command Selection"() -> (w248:i32)
            n130 = property on="Command Selection" class="MCListbox (strict)"("ActiveCell"=w256, "CellBG"=w255, "ActiveCell"=w254, "CellBG"=w253) -> ()  [unwired: 2 in, 2 out]
            n131 = call <vilib>:"WPI_DashboardUpdate RPC Info.vi"("Operation"=w249) -> ("update"=w247:bool, "commands"=w246:string[][])  [unwired: 9 in]
            n132 = property on="Command Selection" class="MCListbox (strict)"("ItemNames"=w246) -> ()  [unwired: 2 in, 2 out]
            n133 = property on="Command Params" class="Tbl (strict)"("Active Cell"=w256, "Cell BG Color"=w255, "Active Cell"=w254, "Cell BG Color"=w253) -> ()  [unwired: 2 in, 2 out]
            n134 = call <vilib>:"WPI_DashboardUpdate Command Params.vi"("Update"=w247, "NewVal"=w248, "Commands"=w246, "Param Tbl"=w245) -> ()  [unwired: 7 in, 1 out]
          }
        }
        n135 = case shown="\"\"" w232 {
          tunnel: "/TestMode/TestProgress" ("Name") -> [w259 _]
          tunnel: "/TestMode/TestProgressText" ("Name") -> [w258 _]
          frame Default {
            n136 = call <vilib>:"NT Read Number.vi"("Name"=w259) -> ("Numeric"=w260:dbl)  [unwired: 9 in, 1 out]
            n137 = call <vilib>:"NT Read String.vi"("Name"=w258) -> ("String"=w261:string)  [unwired: 9 in, 1 out]
            n138 = Bundle("Numeric"=w260, "String"=w261) -> (→"Progress":cluster{"Numeric":dbl, "String":string})  [unwired: 1 in]
          }
          frame "" {
            n139 = property on="Progress" class="Clust (strict)"("Visible"=FALSE) -> ()  [unwired: 2 in, 2 out]
            n140 = local write "Test Name"(u16 0) -> ()
          }
        }
        n141 = call <vilib>:"Connextion Info.vi"() -> ("Connected"=→"NT Connection":bool)  [unwired: 10 in, 1 out]
      }
      event "Test Tree": Value Change {
        # "Show appropriate\ncontrols"
        n142 = event-data() -> ("CtlRef"=w270:refnum<vi>, "NewVal"=w268:string)  [unwired: 1 in]
        n143 = call <vilib>:"WPI_UtilitiesGetTreeIOName.vi"("NewVal"=w268, "TreeControl in"=w270) -> ("I/O Name"=w271:string)  [unwired: 9 in]
        n144 = case shown="\"Analog Out\", \"Motor\", \"PWM\"" w271 {
          selector: w271 -> [_ w278 _ w300 w309 _]
          tunnel: w268 -> [_ _ w297 w299 _ w316]
          tunnel: w267 -> [_ _ _ _ _ w315]
          frame Default {
            w273 = FALSE ("Visible")
            w272 = FALSE ("Visible")
            n145 = property on="Motor" class="Clust (strict)"("Visible"=w272) -> ()  [unwired: 2 in, 2 out]
            n146 = property on="Test Ring" class="Ring (strict)"("Visible"=w272) -> ()  [unwired: 2 in, 2 out]
            n147 = property on="Rev/Fwd" class="Clust (strict)"("Visible"=w273) -> ()  [unwired: 2 in, 2 out]
            n148 = property on="On/Off" class="Bool (strict)"("Visible"=w273) -> ()  [unwired: 2 in, 2 out]
            n149 = property on="Test Slider" class="Slide (strict)"("Visible"=w273) -> ()  [unwired: 2 in, 2 out]
          }
          frame "Analog Out", "Motor", "PWM" {
            w279 = FALSE ("Visible")
            n150 = case shown="\"Analog Out\"" w278 {
              tunnel: [1.0 ("Value") -1.0 ("Value") 0.0 ("Value")] -> w277
              tunnel: [255.0 ("Value") 1.0 ("Value") 5.0 ("Value")] -> w276
              tunnel: [128.0 ("Value") 0.0 ("Value") 0.0 ("Value")] -> w275
              tunnel: [64.0 ("Value") 0.5 ("Value") 1.0 ("Value")] -> w274
              frame "PWM" {
              }
              frame "Motor", Default {
              }
              frame "Analog Out" {
              }
            }
            n151 = property on="Motor" class="Clust (strict)"("Visible"=TRUE) -> ()  [unwired: 2 in, 2 out]
            n152 = property on="Value" class="Slide (strict)"("Value"=w275, "Scale.Minimum"=w277, "Scale.Maximum"=w276, "Scale.Increment"=w274) -> ()  [unwired: 2 in, 2 out]
            n153 = property on="On/Off" class="Bool (strict)"("Visible"=w279) -> ()  [unwired: 2 in, 2 out]
            n154 = property on="Test Slider" class="Slide (strict)"("Visible"=w279) -> ()  [unwired: 2 in, 2 out]
            n155 = property on="Test Ring" class="Ring (strict)"("Visible"=w279) -> ()  [unwired: 2 in, 2 out]
            n156 = property on="Rev/Fwd" class="Clust (strict)"("Visible"=w279) -> ()  [unwired: 2 in, 2 out]
          }
          frame "Servo" {
            w295 = FALSE ("Visible")
            n157 = call <vilib>:"NT Read Number.vi"("Name"=w297) -> ("Numeric"=w296:dbl)  [unwired: 9 in, 1 out]
            n158 = property on="Test Slider" class="Slide (strict)"("Visible"=TRUE, "Scale.Maximum"=170.0 ("Scale.Range:Maximum")) -> ()  [unwired: 2 in, 2 out]
            n159 = local write "Test Slider"(w296) -> ()
            n160 = property on="Motor" class="Clust (strict)"("Visible"=w295) -> ()  [unwired: 2 in, 2 out]
            n161 = property on="Rev/Fwd" class="Clust (strict)"("Visible"=w295) -> ()  [unwired: 2 in, 2 out]
            n162 = property on="On/Off" class="Bool (strict)"("Visible"=w295) -> ()  [unwired: 2 in, 2 out]
            n163 = property on="Test Ring" class="Ring (strict)"("Visible"=w295) -> ()  [unwired: 2 in, 2 out]
          }
          frame "Relay", "Solenoid" {
            w298 = FALSE ("Visible")
            n164 = property on="Motor" class="Clust (strict)"("Visible"=w298) -> ()  [unwired: 2 in, 2 out]
            n165 = property on="Test Slider" class="Slide (strict)"("Visible"=w298) -> ()  [unwired: 2 in, 2 out]
            n166 = Search and Replace String(input string=w299, search string="/Value  **", replace string="/Direction") -> (result string=w305:string)  [unwired: 5 in, 3 out]
            n167 = property on="Test Ring" class="Ring (strict)"("Visible"=w298) -> ()  [unwired: 2 in, 2 out]
            n168 = call <vilib>:"NT Read String.vi"("Name"=w305) -> ("String"=w303:string)  [unwired: 9 in, 1 out]
            n169 = Equal?(x="Both directions", y=w303) -> (x = y?=w301:bool)
            n170 = Not(x=w301) -> (.not. x?=w302:bool)
            n171 = property on="Rev/Fwd" class="Clust (strict)"("Visible"=w301) -> ()  [unwired: 2 in, 2 out]
            n172 = property on="On/Off" class="Bool (strict)"("Visible"=w302, "Caption.Text"=w300) -> ()  [unwired: 2 in, 2 out]
          }
          frame "Compressor", "Digital Out" {
            w308 = FALSE ("Visible")
            # "Get direction and finish"
            n173 = property on="Motor" class="Clust (strict)"("Visible"=w308) -> ()  [unwired: 2 in, 2 out]
            n174 = property on="Test Slider" class="Slide (strict)"("Visible"=w308) -> ()  [unwired: 2 in, 2 out]
            n175 = property on="Test Ring" class="Ring (strict)"("Visible"=w308) -> ()  [unwired: 2 in, 2 out]
            n176 = property on="On/Off" class="Bool (strict)"("Visible"=TRUE, "Caption.Text"=w309) -> ()  [unwired: 2 in, 2 out]
            n177 = property on="Rev/Fwd" class="Clust (strict)"("Visible"=FALSE) -> ()  [unwired: 2 in, 2 out]
          }
          frame "Camera" {
            n178 = call <vilib>:"Get Last Path Segment.vi"("String in"=w316) -> ("String out"=w317:string)  [unwired: 10 in]
            n179 = property on="On/Off" class="Bool (strict)"("Visible"=FALSE) -> ()  [unwired: 2 in, 2 out]
            n180 = property on="Motor" class="Clust (strict)"("Visible"=FALSE) -> ()  [unwired: 2 in, 2 out]
            n181 = property on="Rev/Fwd" class="Clust (strict)"("Visible"=FALSE) -> ()  [unwired: 2 in, 2 out]
            n182 = case shown="\"White Balance  **\"" w317 {
              tunnel: w316 -> [w323 w332 w341 w350 w359 _ w365]
              tunnel: w315 -> [w321 w329 w338 w347 w356 _ _]
              frame "Size  **" {
                n183 = Index Array(array=w321) -> (element=w320:cluster{string[]})  [unwired: 1 in]
                n184 = call <vilib>:"NT Read String.vi"("Name"=w323) -> ("String"=w322:string)  [unwired: 9 in, 1 out]
                n185 = Unbundle(w320) -> (w318:string[])
                n186 = Match First String(2:w318, 3:w322) -> (0:w319:i32)  [unwired: 1 out]
                n187 = property on="Test Ring" class="Ring (strict)"("Value"=w319, "Strings []"=w318) -> ()  [unwired: 2 in, 2 out]
                n188 = property on="Test Ring" class="Ring (strict)"("Visible"=TRUE) -> ()  [unwired: 2 in, 2 out]
                n189 = property on="Test Slider" class="Slide (strict)"("Visible"=FALSE) -> ()  [unwired: 2 in, 2 out]
              }
              frame "White Balance  **" {
                n190 = Index Array(array=w329, index=1) -> (element=w330:cluster{string[]})
                n191 = call <vilib>:"NT Read String.vi"("Name"=w332) -> ("String"=w331:string)  [unwired: 9 in, 1 out]
                n192 = Unbundle(w330) -> (w327:string[])
                n193 = Match First String(2:w327, 3:w331) -> (0:w326:i32)  [unwired: 1 out]
                n194 = property on="Test Ring" class="Ring (strict)"("Value"=w326, "Strings []"=w327) -> ()  [unwired: 2 in, 2 out]
                n195 = property on="Test Ring" class="Ring (strict)"("Visible"=TRUE) -> ()  [unwired: 2 in, 2 out]
                n196 = property on="Test Slider" class="Slide (strict)"("Visible"=FALSE) -> ()  [unwired: 2 in, 2 out]
              }
              frame "Exposure  **" {
                n197 = Index Array(array=w338, index=2) -> (element=w339:cluster{string[]})
                n198 = call <vilib>:"NT Read String.vi"("Name"=w341) -> ("String"=w340:string)  [unwired: 9 in, 1 out]
                n199 = Unbundle(w339) -> (w335:string[])
                n200 = Match First String(2:w335, 3:w340) -> (0:w336:i32)  [unwired: 1 out]
                n201 = property on="Test Ring" class="Ring (strict)"("Value"=w336, "Strings []"=w335) -> ()  [unwired: 2 in, 2 out]
                n202 = property on="Test Ring" class="Ring (strict)"("Visible"=TRUE) -> ()  [unwired: 2 in, 2 out]
                n203 = property on="Test Slider" class="Slide (strict)"("Visible"=FALSE) -> ()  [unwired: 2 in, 2 out]
              }
              frame "Exposure Priority  **" {
                n204 = Index Array(array=w347, index=3) -> (element=w348:cluster{string[]})
                n205 = call <vilib>:"NT Read String.vi"("Name"=w350) -> ("String"=w349:string)  [unwired: 9 in, 1 out]
                n206 = Unbundle(w348) -> (w344:string[])
                n207 = Match First String(2:w344, 3:w349) -> (0:w345:i32)  [unwired: 1 out]
                n208 = property on="Test Ring" class="Ring (strict)"("Value"=w345, "Strings []"=w344) -> ()  [unwired: 2 in, 2 out]
                n209 = property on="Test Ring" class="Ring (strict)"("Visible"=TRUE) -> ()  [unwired: 2 in, 2 out]
                n210 = property on="Test Slider" class="Slide (strict)"("Visible"=FALSE) -> ()  [unwired: 2 in, 2 out]
              }
              frame "Color Enable  **" {
                n211 = Index Array(array=w356, index=4) -> (element=w357:cluster{string[]})
                n212 = call <vilib>:"NT Read String.vi"("Name"=w359) -> ("String"=w358:string)  [unwired: 9 in, 1 out]
                n213 = Unbundle(w357) -> (w353:string[])
                n214 = Match First String(2:w353, 3:w358) -> (0:w354:i32)  [unwired: 1 out]
                n215 = property on="Test Ring" class="Ring (strict)"("Value"=w354, "Strings []"=w353) -> ()  [unwired: 2 in, 2 out]
                n216 = property on="Test Ring" class="Ring (strict)"("Visible"=TRUE) -> ()  [unwired: 2 in, 2 out]
                n217 = property on="Test Slider" class="Slide (strict)"("Visible"=FALSE) -> ()  [unwired: 2 in, 2 out]
              }
              frame Default {
                n218 = property on="Test Ring" class="Ring (strict)"("Visible"=FALSE) -> ()  [unwired: 2 in, 2 out]
                n219 = property on="Test Slider" class="Slide (strict)"("Visible"=FALSE) -> ()  [unwired: 2 in, 2 out]
              }
              frame "Brightness  **", "Color Level  **", "Compression  **", "FPS  **", "Sharpness  **" {
                n220 = call <vilib>:"NT Read Number.vi"("Name"=w365) -> ("Numeric"=w364:dbl)  [unwired: 9 in, 1 out]
                n221 = local write "Test Slider"(w364) -> ()
                n222 = property on="Test Slider" class="Slide (strict)"("Visible"=TRUE, "Scale.Maximum"=100.0 ("Scale.Range:Maximum")) -> ()  [unwired: 2 in, 2 out]
                n223 = property on="Test Ring" class="Ring (strict)"("Visible"=FALSE) -> ()  [unwired: 2 in, 2 out]
              }
            }
          }
        }
        n224 = property on="Progress" class="Clust (strict)"("Visible"=FALSE) -> ()  [unwired: 2 in, 2 out]
      }
      event "Test Name": Mouse Enter {
        # "Populate the ring with the list of tests"
        n225 = event-data() -> ()  [unwired: 1 in, 1 out]
        n226 = call <vilib>:"NT Read String Array.vi"("Name"="/TestMode/TestList") -> ("String Array"=w374:string[])  [unwired: 9 in, 1 out]
        n227 = Build Array (concatenate)("Select the test to run...", w374) -> (w373:string[])
        n228 = property on="Test Name" class="Ring (strict)"("Strings []"=w373) -> ()  [unwired: 2 in, 2 out]
      }
      event "Test Name": Value Change {
        w377 = FALSE ("Visible")
        # "Tell the robot the test name to run"
        n229 = event-data() -> ("NewVal"=w381:u16)  [unwired: 1 in]
        n230 = property on="Test Name" class="Ring (strict)"() -> ("Strings []"=w382:string[])  [unwired: 2 in, 2 out]
        n231 = local write "Progress"(T7 {"Test Progress"=0, "Test Progress Text"=""} ("Progress")) -> ()
        n232 = Index Array(array=w382, index=w381) -> (element=w380:string)
        n233 = call <vilib>:"NT Write String.vi"("String"=w380, "Name"="/TestMode/TestName") -> ()  [unwired: 9 in, 1 out]
        n234 = property on="Progress" class="Clust (strict)"("Visible"=TRUE) -> ()  [unwired: 2 in, 2 out]
        n235 = property on="Motor" class="Clust (strict)"("Visible"=w377) -> ()  [unwired: 2 in, 2 out]
        n236 = property on="Test Slider" class="Slide (strict)"("Visible"=w377) -> ()  [unwired: 2 in, 2 out]
        n237 = property on="On/Off" class="Bool (strict)"("Visible"=w377) -> ()  [unwired: 2 in, 2 out]
        n238 = property on="Rev/Fwd" class="Clust (strict)"("Visible"=w377) -> ()  [unwired: 2 in, 2 out]
        n239 = property on="Test Ring" class="Ring (strict)"("Visible"=w377) -> ()  [unwired: 2 in, 2 out]
      }
      event "Select Auto": Mouse Enter {
        # "Populate the combo box with the list of autonomous options"
        n240 = event-data() -> ()  [unwired: 1 in, 1 out]
        n241 = call <vilib>:"NT Read String Array.vi"("Name"="Auto List") -> ("String Array"=w384:string[])  [unwired: 9 in, 1 out]
        n242 = property on="Select Auto" class="CmbBox"("Strings[]"=w384) -> ()  [unwired: 2 in, 2 out]
      }
      event "Select Auto": Value Change {
        # "User modified the Auto Selection. Write to NT variable so robot knows."
        n243 = event-data() -> ("NewVal"=w388:string)  [unwired: 1 in]
        n244 = call <vilib>:"NT Write String.vi"("String"=w388, "Name"="Auto Selector") -> ()  [unwired: 9 in, 1 out]
      }
      event "Command Selection": Value Change {
        # "Get the params and show in table"
        n245 = event-data() -> ("NewVal"=w395:i32)  [unwired: 1 in]
        n246 = property on="Command Selection" class="MCListbox (strict)"() -> ("ItemNames"=w393:string[][])  [unwired: 2 in, 2 out]
        n247 = call <vilib>:"WPI_DashboardUpdate Command Params.vi"("NewVal"=w395, "Commands"=w393, "Param Tbl"=w394) -> ()  [unwired: 8 in, 1 out]
      }
      event "Execute Command": Value Change {
        # "Started one, Unique ID holds\nresponse"
        n248 = event-data() -> ()  [unwired: 1 in, 1 out]
        n249 = property on="Command Selection" class="MCListbox (strict)"() -> ("ItemNames"=w407:string[][])  [unwired: 2 in, 2 out]
        n250 = Index Array(array=w407, index (row)="Command Selection", index (col)=0) -> (element=w405:string)
        n251 = call <vilib>:"Invoke Commands.vi"("Command Params"="Command Params", "Function Name"=w405) -> ("Params"=w401:u8, "Started"=w400:bool)  [unwired: 7 in, 1 out]
        n252 = Array Subset(array="Command Params", length (row)=w401) -> (w402:string[][])  [unwired: 3 in]
        n253 = Select(t="Executing" ("Cmd Status"), s=w400, f="" ("Cmd Status")) -> (s? t:f=→"Cmd Status":string)
      }
      event "Command Selection": Double Click {
        n254 = event-data() -> ("Row"=w417:i32)  [unwired: 1 in]
        n255 = property on="Command Selection" class="MCListbox (strict)"() -> ("ItemNames"=w420:string[][])  [unwired: 2 in, 2 out]
        n256 = local read "Command Params"() -> (w415:string[][])
        n257 = Index Array(array=w420, index (row)=w417, index (col)=0) -> (element=w418:string)
        n258 = call <vilib>:"Invoke Commands.vi"("Command Params"=w415, "Function Name"=w418) -> ("Params"=w414:u8, "Started"=w409:bool)  [unwired: 7 in, 1 out]
        n259 = Array Subset(array=w415, length (row)=w414) -> (w413:string[][])  [unwired: 3 in]
        n260 = Select(t="Executing" ("Cmd Status"), s=w409, f="" ("Cmd Status")) -> (s? t:f=w410:string)
        n261 = local write "Cmd Status"(w410) -> ()
      }
      event "CheckList": Double Click {
        # "Shift clears all"
        # "Update symbols on the listbox"
        n262 = event-data() -> ("PlatMods.Shift"=w423:bool, "Row"=w425:i32)  [unwired: 1 in]
        n263 = case shown="True" w423 {
          tunnel: w425 -> [w429 _]
          tunnel: 1 -> [w428 _]
          frame False {
            n264 = property on="CheckList" class="LstBox (strict)"() -> ("Item Symbols"=w427:i32[])  [unwired: 2 in, 2 out]
            n265 = Replace Array Subset(array=w427, new element=w428, index=w429) -> (w426:i32[])
            n266 = property on="CheckList" class="LstBox (strict)"("Item Symbols"=w426) -> ()  [unwired: 2 in, 2 out]
          }
          frame True {
            w430 = 0 ("Top Row")
            n267 = property on="CheckList" class="LstBox (strict)"() -> ("Number of Rows"=w432:u32)  [unwired: 2 in, 2 out]
            n268 = Initialize Array(0, w432) -> (w431:i32[])
            n269 = property on="CheckList" class="LstBox (strict)"("Top Row"=w430, "Value"=w430, "Item Symbols"=w431) -> ()  [unwired: 2 in, 2 out]
          }
        }
      }
      event "CheckList": Key Down {
        # "Update symbols on the listbox\nLeft and right keys check and uncheck"
        n270 = event-data() -> ("VKey"=w437:T22)  [unwired: 1 in]
        n271 = case shown="\"Left\", \"Right\"" w437 {
          selector: w437 -> [w442 _]
          tunnel: eventvkey."Left" ("VKey") -> [w440 _]
          frame "Left", "Right" {
            n272 = Equal?(x=w440, y=w442) -> (x = y?=w441:bool)
            n273 = Select(t=0, s=w441, f=1) -> (s? t:f=w443:i32)
            n274 = property on="CheckList" class="LstBox (strict)"() -> ("Item Symbols"=w446:i32[])  [unwired: 2 in, 2 out]
            n275 = Replace Array Subset(array=w446, new element=w443, index="CheckList") -> (w445:i32[])
            n276 = property on="CheckList" class="LstBox (strict)"("Item Symbols"=w445) -> ()  [unwired: 2 in, 2 out]
          }
          frame Default {
          }
        }
      }
      event "DB Camera Config": Value Change {
        # "Show or hide the cluster of controls, store in ini file"
        n277 = event-data() -> ("NewVal"=w451:bool)  [unwired: 1 in]
        n278 = case shown="False" w451 {
          tunnel: w450 -> [w460 _]
          tunnel: [w453 w471] -> w449
          tunnel: w448 -> [w452 w471]
          frame False {
            w467 = "Camera"
            w470 = FALSE ("Visible")
            n279 = local read "Camera Settings"() -> (w459:T2)
            n280 = Index Array(array=w460) -> (element=w463:cluster{string[]})  [unwired: 1 in]
            n281 = Unbundle(w459) -> ("Frame Rate"=w458:i32, "Compression"=w457:i32, "Size"=w461:u16)
            n282 = Unbundle(w463) -> (w462:string[])
            n283 = Index Array(array=w462, index=w461) -> (element=w456:string)
            n284 = call-poly <vilib>:"Write Key.vi"("section"=w467, "value"=w456, "key"="Size", "refnum"=w452) -> ("refnum out"=w469:T20)  [unwired: 2 in, 5 out]
            n285 = call-poly <vilib>:"Write Key.vi"("section"=w467, "value"=w458, "key"="FrameRate", "refnum"=w469) -> ("refnum out"=w468:T20)  [unwired: 1 in, 6 out]
            n286 = property on="Camera Settings" class="Clust (strict)"("Visible"=w470) -> ()  [unwired: 2 in, 2 out]
            n287 = local write "DB Camera Config"(w470) -> ()
            n288 = call-poly <vilib>:"Write Key.vi"("section"=w467, "value"=w457, "key"="Compression", "refnum"=w468) -> ("refnum out"=w454:T20)  [unwired: 1 in, 6 out]
            n289 = call <vilib>:"Close Config Data.vi"("refnum"=w454) -> ("file path"=w455:path)  [unwired: 2 in, 8 out]
            n290 = call <vilib>:"Open Config Data.vi"("configuration file path"=w455) -> ("refnum"=w453:T20)  [unwired: 8 in, 2 out]
          }
          frame True {
            n291 = property on="Camera Settings" class="Clust (strict)"("Visible"=TRUE) -> ()  [unwired: 2 in, 2 out]
          }
        }
      }
      event "Camera Settings": Value Change {
        # "Update summary string when any elements of DB camera change"
        n292 = event-data() -> ("NewVal"=w485:T2)  [unwired: 1 in]
        n293 = Index Array(array=w481) -> (element=w480:cluster{string[]})  [unwired: 1 in]
        n294 = Unbundle(w485) -> ("Frame Rate"=w476:i32, "Compression"=w475:i32, "Size"=w478:u16)
        n295 = Unbundle(w480) -> (w479:string[])
        n296 = Index Array(array=w479, index=w478) -> (element=w477:string)
        n297 = Format Into String(format string="%s   %dfps   %d%%", w477, w476, w475) -> (resulting string=w482:string)  [unwired: 2 in, 1 out]
        n298 = Build Array(w482) -> (w483:string[])
        n299 = property on="DB Camera Config" class="Bool (strict)"("Strings [4]"=w483) -> ()  [unwired: 2 in, 2 out]
      }
      event "Motor.Enable": Value Change {
        # "When the test mode otor enable helper is set, update that\ntree row item's value"
        n300 = event-data() -> ("NewVal"=w492:bool)  [unwired: 1 in]
        n301 = Unbundle("Motor") -> ("Value"=w491:dbl)  [unwired: 1 out]
        n302 = Select(t=w491, s=w492, f=0.0) -> (s? t:f=w489:dbl)
        n303 = call <vilib>:"NT Write Number.vi"("Numeric"=w489, "Name"=w488) -> ()  [unwired: 9 in, 1 out]
      }
      event "Test Slider": Value Change {
        # "When the test mode slider helper is set, update that\ntree row item's value"
        n304 = event-data() -> ("NewVal"=w496:dbl)  [unwired: 1 in]
        n305 = call <vilib>:"NT Write Number.vi"("Numeric"=w496, "Name"=w497) -> ()  [unwired: 9 in, 1 out]
      }
      event "On/Off": Value Change {
        # "When the test mode on/off helper value is set, update that\ntree row item's value"
        n306 = event-data() -> ("NewVal"=w502:bool)  [unwired: 1 in]
        n307 = Boolean To (0,1)(Boolean=w502) -> (0, 1=w501:i16)
        n308 = call <vilib>:"NT Write Number.vi"("Numeric"=w501, "Name"=w500) -> ()  [unwired: 9 in, 1 out]
      }
      event "Rev/Fwd": Value Change {
        # "When the test mode helper value for relays is set, update that\ntree row item's value"
        n309 = event-data() -> ("NewVal.Forward"=w511:bool, "NewVal.Reverse"=w510:bool)  [unwired: 1 in]
        n310 = Boolean To (0,1)(Boolean=w511) -> (0, 1=w507:i16)
        n311 = Boolean To (0,1)(Boolean=w510) -> (0, 1=w509:i16)
        n312 = Negate(x=w509) -> (-x=w508:i16)
        n313 = Add(x=w507, y=w508) -> (x+y=w506:i16)
        n314 = call <vilib>:"NT Write Number.vi"("Numeric"=w506, "Name"=w505) -> ()  [unwired: 9 in, 1 out]
      }
      event "Test Ring": Value Change {
        # "When a test mode helper value is selected from the ring,\nset the tree item's variable to the string value"
        n315 = event-data() -> ("NewVal"=w516:u16)  [unwired: 1 in]
        n316 = property on="Test Ring" class="Ring (strict)"() -> ("Strings []"=w517:string[])  [unwired: 2 in, 2 out]
        n317 = Index Array(array=w517, index=w516) -> (element=w515:string)
        n318 = call <vilib>:"NT Write String.vi"("String"=w515, "Name"=w514) -> ()  [unwired: 9 in, 1 out]
      }
      event "Rec Mode": Value Change {
        # "Update globals for recording mode and path to read log from.\nClear when logging and let NetworkTables set path for vision to\nuse."
        n319 = event-data() -> ("NewVal"=w529:enum32{"Stop", "Record", "Playback"})  [unwired: 1 in]
        n320 = global write "WPI_DashboardLogging Global.vi" "Logging Filename"(path "") -> ()
        n321 = global write "WPI_DashboardLogging Global.vi" "Recording"(w529) -> ()
        n322 = case shown="\"Playback\"" w529 {
          tunnel: w528 -> [_ w531 w540]
          tunnel: [_ _ w539] -> w525
          tunnel: [_ _ w538] -> _
          tunnel: w523 -> [_ _ w536]
          tunnel: cluster{i32, i32} {-250, 170} -> [_ _ w535]
          tunnel: [_ _ T23 {"Image Size"=TRUE, "Image Type"=TRUE, "Pixel Value"=TRUE, "ROI Information"=TRUE, "Zoom Factor"=FALSE} ("Image Information Shown:All Elements")] -> w521
          tunnel: [_ _ TRUE ("Zoom Factor")] -> w520
          tunnel: w519 -> [_ _ w532]
          frame Default {
          }
          frame "Stop", "Record" {
            # "Place Window too"
            n323 = invoke class="VI" method="FP.Close"(reference=w531) -> (reference out=w530:refnum<vi>)  [unwired: 2 in, 2 out]
            n324 = invoke class="VI" method="Abort VI"(reference=w530) -> ()  [unwired: 2 in, 3 out]
          }
          frame "Playback" {
            n325 = call "Open Playback Panel.vi"("Offset"=w535, "DB VI Ref"=w536, "Playback in"=w540) -> ("Playback out"=w537:refnum<vi>)  [unwired: 8 in]
            n326 = register-events(w537, w532) -> (reference out=w539:refnum<event-registration>, error out=w538:errorcluster)  [unwired: 2 in]
          }
        }
        n327 = property on="Camera Image" class="ImageControl"("Image Information Shown"=w521, "Image Information Visible"=w520) -> ()  [unwired: 2 in, 2 out]
        n328 = call <vilib>:"WPI_DashboardNT Log FieldName Cache.vi"("Operation"=enum16{"Lookup/Add", "Index", "Clear"}."Clear") -> ()  [unwired: 8 in, 3 out]
      }
      event Panel Close {
        w542 = enum32{"Stop", "Record", "Playback"}."Stop" ("Rec Mode")
        # "Playback window has been closed, abort"
        n329 = event-data() -> ()  [unwired: 1 in, 4 out]
        n330 = local write "Rec Mode"(w542) -> ()
        n331 = global write "WPI_DashboardLogging Global.vi" "Recording"(w542) -> ()
      }
      event Panel Close {
        # "Abort playback window and ourself"
        n332 = event-data() -> ()  [unwired: 1 in, 4 out]
        n333 = invoke class="VI" method="FP.Close"(reference=w548) -> (reference out=w547:refnum<vi>)  [unwired: 2 in, 2 out]
        n334 = invoke class="VI" method="Abort VI"(reference=w547) -> (error out=w546:errorcluster)  [unwired: 2 in, 2 out]
        n335 = invoke class="VI" method="Abort VI"(error in=w546) -> ()  [unwired: 2 in, 3 out]
      }
      event User Event {
        n336 = event-data() -> ("IDs"=w556:cluster{"RPC field ID":u16, "Unique ID":u16}, "String"=w555:string)  [unwired: 1 in]
        n337 = Bundle("IDs"=w556, "String"=w555) -> (w554:T9)  [unwired: 1 in]
        n338 = call <vilib>:"Retrieve RPC Response.vi"("RPC Response"=w554) -> ("Output"=w551:string[][])  [unwired: 10 in]
        n339 = Build Array (concatenate)(w549, w551) -> (w550:string[][])
        n340 = local write "Command Params"(w550) -> ()
        n341 = local write "Cmd Status"("" ("Cmd Status")) -> ()
      }
      event "Vision": Value Change {
        # "Enable/Disable Compression slider.\nHW USB is hard-coded into the camera"
        n342 = event-data() -> ("NewVal"=w563:u16)  [unwired: 1 in]
        n343 = Equal?(x=w563, y=u32 2 ("milliseconds to wait")) -> (x = y?=w561:bool)
        n344 = Select(t=T24."Disabled and Grayed Out" ("Disabled"), s=w561, f=T24."Enabled" ("Disabled")) -> (s? t:f=w558:T24)
        n345 = property on="Compression" class="Slide (strict)"("DisabledEnum"=w558) -> ()  [unwired: 2 in, 2 out]
      }
      event "Tree": Double Click {
        n346 = event-data() -> ("PlatMods"=w568:T27, "Tag"=w567:string)  [unwired: 1 in]
        n347 = Unbundle(w568) -> ("Shift"=w566:bool)  [unwired: 4 out]
        n348 = Not(x=w566) -> (.not. x?=w565:bool)
        n349 = call <vilib>:"NT Update Persistence.vi"("Persistence"=w565, "Name"=w567) -> ()  [unwired: 9 in, 1 out]
      }
    }
  }
  n350 = while {
    tunnel: w53 -> [w572]
    i -> [w575]
    stop <- FALSE stop-if-true
    n351 = Wait (ms)(milliseconds to wait=u32 100) -> ()  [unwired: 1 out]
    n352 = case shown="\"Playback\"" "Rec Mode" {
      tunnel: w575 -> [_ _ w590]
      tunnel: [u32 2829099 ("Base Color") u32 11141120 ("Target Color") w579] -> w571
      frame "Stop", Default {
        # "Reset the color, extra updates don't cost much"
      }
      frame "Record" {
      }
      frame "Playback" {
        # "Playback"
        n353 = Quotient & Remainder(x=w590, y=u32 50 ("milliseconds to wait")) -> (x-y*floor(x/y)=w586:u32)  [unwired: 1 out]
        n354 = Divide(x=w586, y=u32 50 ("milliseconds to wait")) -> (x/y=w583:dbl)
        n355 = Multiply(x=6.283185307179586, y=w583) -> (x*y=w588:dbl)
        n356 = Sine(x=w588) -> (sin(x)=w587:dbl)
        n357 = Absolute Value(x=w587) -> (abs(x)=w580:dbl)
        n358 = call "Interpolate RGB Color.vi"("Proportion"=w580, "Target Color"=u32 30976, "Base Color"=u32 2829099) -> ("Result Color"=w579:u32)  [unwired: 8 in]
      }
    }
    n359 = property class="Pane"(reference=w572, "PaneColor"=w571) -> ()  [unwired: 1 in, 2 out]
  }
  n360 = local write "Dashboard Tab"(T1."Drive" ("Dashboard Tab")) -> ()
  n361 = property on="On/Off" class="Bool (strict)"("Visible"=w21) -> ()  [unwired: 2 in, 2 out]
  n362 = property on="Motor" class="Clust (strict)"("Visible"=w21) -> ()  [unwired: 2 in, 2 out]
  n363 = property on="Progress" class="Clust (strict)"("Visible"=w21) -> ()  [unwired: 2 in, 2 out]
  n364 = property on="Test Ring" class="Ring (strict)"("Visible"=w21) -> ()  [unwired: 2 in, 2 out]
  n365 = property on="Rev/Fwd" class="Clust (strict)"("Visible"=w21) -> ()  [unwired: 2 in, 2 out]
  n366 = property on="Camera Settings" class="Clust (strict)"("Visible"=w21) -> ()  [unwired: 2 in, 2 out]
  n367 = while {
    tunnel: u16 1741 ("timeout ms (25000)") -> [w592]
    stop <- FALSE stop-if-true
    n368 = TCP Create Listener(10:w592) -> (0:w591:errorcluster, 3:w593:refnum<k5>)  [unwired: 4 in, 1 out]
    n369 = case shown="No Error" w591 {
      selector: w591 -> [w595 _]
      tunnel: w593 -> [w596 _]
      frame No Error {
        n370 = while {
          tunnel: w596 -> [w599]
          tunnel: w595 -> [w598]
          stop <- FALSE stop-if-true
          n371 = TCP Wait On Listener(8:w598, 11:w599) -> (0:w600:errorcluster, 4:w601:refnum<k5>)  [unwired: 2 in, 3 out]
          n372 = local write "TCP"(w601) -> ()
          n373 = case shown="No Error" w600 {
            frame No Error {
            }
            frame Error {
              n374 = Wait (ms)(milliseconds to wait=u32 1000) -> ()  [unwired: 1 out]
            }
          }
        }
      }
      frame Error {
        n375 = Wait (ms)(milliseconds to wait=u32 1000) -> ()  [unwired: 1 out]
      }
    }
  }
  n376 = local write "DB Camera Config"(w21) -> ()
  n377 = local write "Command Params"(string[][] [] ("Command Params")) -> ()
  n378 = global write "WPI_DashboardLogging Global.vi" "Recording"(w47) -> ()
  n379 = local write "Command Selection"(u16 0 ("milliseconds to wait")) -> ()
  n380 = local write "Rec Mode"(w47) -> ()
